vi "实验2-2（全局变量）.vi"() -> ()   [LabVIEW 2018]
panel:
  in  "停止":bool
  in  "数值":dbl
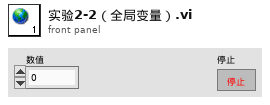
[diagram p1: front panel]
diagram:
